vi "Initialize.vi"(8 "error in":errorcluster, 11 "Shared Resources in":refnum<class "Shared Resources.lvclass">) -> (0 "error out":errorcluster, 3 "Shared Resources out":refnum<class "Shared Resources.lvclass">)   [LabVIEW 2020, in "AIM ARINC 429 Engine.lvlib" / "Implementation.lvlib" / "Shared Resources.lvclass"]
uses:
  Shared Resources.lvclass
  Shared Resources.lvclass/Shared Resources.ctl
  <instrlib>/AIM GmbH/ARINC-429/subvi/Error Converter (ErrCode or Status).vi
  <instrlib>/AIM GmbH/ARINC-429/subvi/Get Library Path.vi
  <instrlib>/AIM GmbH/ARINC-429/VIs/Library/Api429Lib Error Desc Get.vi
  <instrlib>/AIM GmbH/ARINC-429/subvi/Get Error Number Offset.vi
  <vilib>/Utility/error.llb/Error Cluster From Error Code.vi
  Hardware API/AIM ARINC 429 Hardware API.lvlib
  <instrlib>/AIM GmbH/ARINC-429/AIM429LV.lvlib
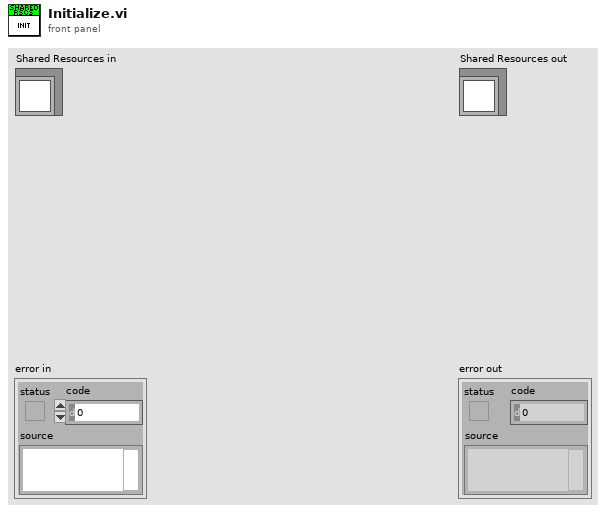
[diagram p1: front panel]
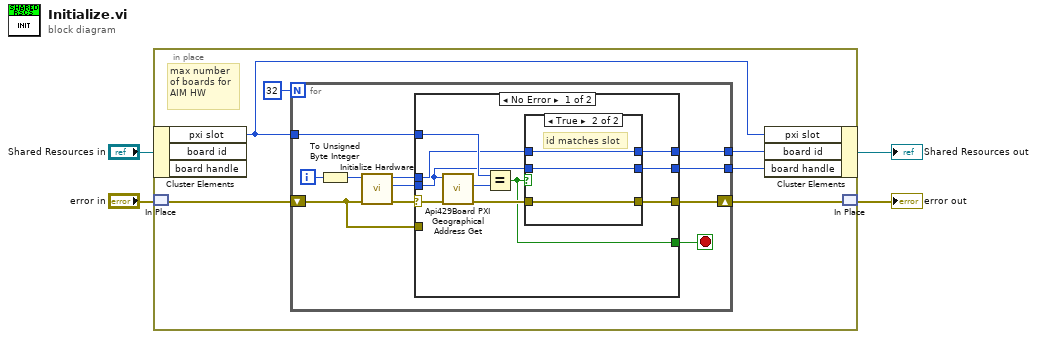
[diagram p0: block diagram]
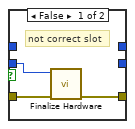
[diagram p2: hidden frame]
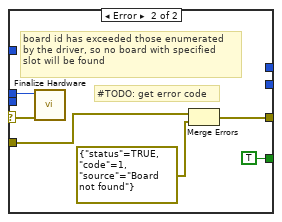
[diagram p3: hidden frame]
diagram:
  n1 = in-place {
    # "max number\nof boards for\nAIM HW"
    n2 = in-place-cluster #1("Shared Resources in") -> ("pxi slot"=w5:u8)  [unwired: 2 out]
    n3 = in-place-match #2("error in") -> (w10:errorcluster)
    n4 = for {
      N: 32 -> [_]
      shift-right: [w16] -> w9
      shift-left: w10 -> [w11]
      tunnel: w5 -> [w17]
      tunnel: [w14] -> w7
      tunnel: [w13] -> w6
      i -> [w21]
      stop <- w12 stop-if-true
      n5 = To Unsigned Byte Integer(number=w21) -> (unsigned 8bit integer=w20:u8)
      n6 = call "Initialize Hardware.vi"("error in"=w11, "board identifier in"=w20) -> ("error out"=w19:errorcluster, "module handle out"=w18:u8, "board identifier out"=w15:u8)  [unwired: 7 in]
      n7 = case shown="No Error" w19 {
        selector: w19 -> [w31 w43]
        tunnel: w18 -> [w28 _]
        tunnel: w17 -> [w29 _]
        tunnel: [w25 w38] -> w16
        tunnel: w15 -> [w24 w42]
        tunnel: [w27 _] -> w14
        tunnel: [w23 _] -> w13
        tunnel: [w22 TRUE] -> w12
        tunnel: w11 -> [_ w40]
        frame No Error {
          n8 = call <instrlib>:"Api429Board PXI Geographical Address Get.vi"("error in (no error)"=w31, "boardHandle"=w28) -> ("error out"=w26:errorcluster, "pxiSlotGeographicalAddress out"=w30:u32)  [unwired: 8 in]
          n9 = Equal?(x=w29, y=w30) -> (x = y?=w22:bool)
          n10 = case shown="True" w22 {
            tunnel: w28 -> [w33 w37]
            tunnel: [_ w37] -> w27
            tunnel: w26 -> [w34 w36]
            tunnel: [w32 w36] -> w25
            tunnel: w24 -> [_ w35]
            tunnel: [_ w35] -> w23
            frame False {
              # "not correct slot"
              n11 = call "Finalize Hardware.vi"("error in"=w34, "board identifier"=w33) -> ("error out"=w32:errorcluster)  [unwired: 9 in]
            }
            frame True {
              # "id matches slot"
            }
          }
        }
        frame Error {
          # "#TODO: get error code"
          # "board id has exceeded those enumerated\nby the driver, so no board with specified\nslot will be found"
          n12 = call "Finalize Hardware.vi"("error in"=w43, "board identifier"=w42) -> ()  [unwired: 9 in, 1 out]
          n13 = Merge Errors(w40, errorcluster {"status"=TRUE, "code"=1, "source"="Board not found"} ("error in (no error)")) -> (w38:errorcluster)
        }
      }
    }
    n14 = in-place-cluster #1("pxi slot"=w5, "board id"=w6, "board handle"=w7) -> (→"Shared Resources out":refnum<class "Shared Resources.lvclass">)
    n15 = in-place-match #2(w9) -> (→"error out":errorcluster)
  }
